vi "testGetPathOfTestMonitor.vi"(8 "error in (no error)":errorcluster) -> (0 "error out":errorcluster)   [LabVIEW 2018]
uses:
  <vilib>/addons/_JKI Toolkits/Caraya/classes/Assert/Assert True.vi
  <vilib>/addons/_JKI Toolkits/Caraya/classes/Assert/Assert Equal Value_Variant.vi
  <vilib>/addons/_JKI Toolkits/Caraya/classes/Test/Test.lvclass
  <vilib>/addons/_JKI Toolkits/Caraya/classes/Assert/Assert.lvclass
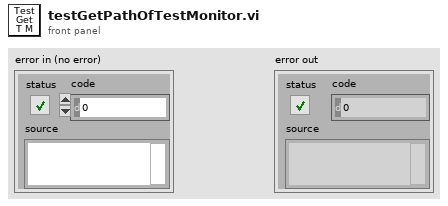
[diagram p1: front panel]
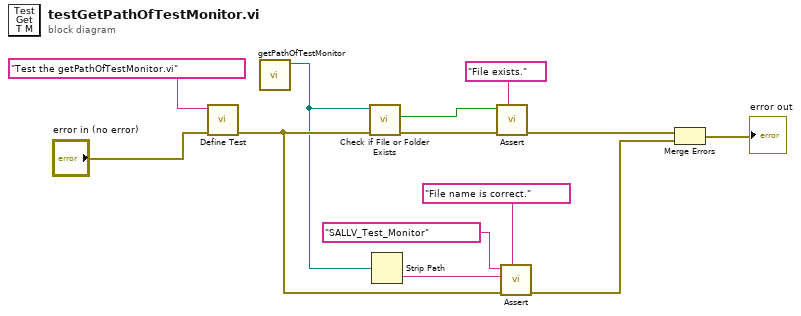
[diagram p0: block diagram]
diagram:
  n1 = call <vilib>:"Define Test.vi"("error in (no error)"="error in (no error)", "Label (VI Title)"="Test the getPathOfTestMonitor.vi") -> ("error out"=w8:errorcluster)  [unwired: 9 in]
  n2 = call "getPathOfTestMonitor.vi"() -> ("testMonitorPath"=w1:path)  [unwired: 11 in]
  n3 = call <vilib>:"Check if File or Folder Exists.vi"("error in (no error)"=w8, "path"=w1) -> ("error out"=w11:errorcluster, "file or folder exists?"=w10:bool)  [unwired: 7 in, 1 out]
  n4 = Strip Path(path=w1) -> (name=w7:string)  [unwired: 1 out]
  n5 = call-poly <vilib>:"Assert.vi"("Label"="File exists.", "error in (no error)"=w11, "True?"=w10) -> ("error out"=w4:errorcluster)  [unwired: 8 in]
  n6 = call-poly <vilib>:"Assert.vi"("Label"="File name is correct.", "error in (no error)"=w8, "Y"=w7, "X"="SALLV_Test_Monitor") -> ("error out"=w3:errorcluster)  [unwired: 7 in]
  n7 = Merge Errors(w4, w3) -> (→"error out":errorcluster)
